vi "Normalize Polynomial.vi"(0 "Numerator":dbl[](array[numeric])=[1.0] format="%.2f", 1 "Denominator":dbl[](array[numeric]) format="%.2f") -> (2 "Numerator new":dbl[](array[numeric]) format="%.2f", 3 "Denominator new":dbl[](array[numeric]) format="%.2f", 4 "additive constant":dbl format="%.2f", 5 "error":i32)   [LabVIEW 2017, in "NI_AdvCtrl_continuous linear.lvlib"]
doc: "LabVIEW no longer supports this VI. You can obtain similar functionality by installing the LabVIEW Simulation Module."
uses:
  <vilib>/addons/control/advanced/NI_AdvCtrl_continuous linear.lvlib
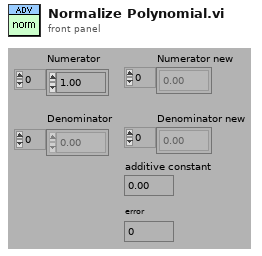
[diagram p1: front panel]
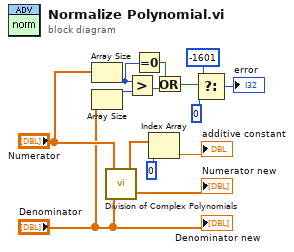
[diagram p0: block diagram]
diagram:
  n1 = Array Size(array="Numerator") -> (size(s)=w1:i32)
  n2 = Array Size(array="Denominator") -> (size(s)=w10:i32)
  n3 = call <vilib>:"Division of Complex Polynomials.vi"("Q"="Denominator", "P"="Numerator") -> ("Rest"=→"Numerator new":cdb[], "P/Q"=w12:cdb[])
  n4 = Greater?(x=w1, y=w10) -> (0:w7:bool)
  n5 = Equal To 0?(x=w1) -> (x = 0?=w2:bool)
  n6 = Index Array(array=w12, index=0) -> (element=→"additive constant":cdb)
  n7 = Or(x=w2, y=w7) -> (x .or. y?=w3:bool)
  n8 = Select(t=-1601 ("error"), s=w3, f=0 ("error")) -> (s? t:f=→"error":i32)
  "Denominator new" <- "Denominator"
